vi "Clustering.vi"() -> ()   [LabVIEW 2014]
uses:
  <vilib>/Analysis/Matrix/Datatypes/RealMatrix.ctl
  <vilib>/Analysis/baseanly.llb/Real A x B.vi
  <vilib>/Utility/file.llb/Read From Spreadsheet File (DBL).vi
  <vilib>/Analysis/Matrix/Numeric/Conversions/Matrix To Array - RM.vi
  <vilib>/Utility/file.llb/Read From Spreadsheet File (I64).vi
  <vilib>/Analysis/NI_AALBase.lvlib
  <vilib>/Analysis/Matrix/NI_Matrix.lvlib
panel:
  out "TFD Clustering":i32[](array[numeric])
  out "Centroids of TFD":T1
  out "Centroids of Z (KLD)":T1
  out "Z Clustering (KDL)":i32[](array[numeric])
  out "Centroids of Z (EUC)":T1
  out "Z Clustering (EUC)":i32[](array[numeric])
  out "Centroids of Matrix A":T1
  out "mixing_A Clustering":i32[](array[numeric])
  in  "mixing_A":path
  in  "Selected":path
  in  "inverse_W":path
  in  "STFT":path
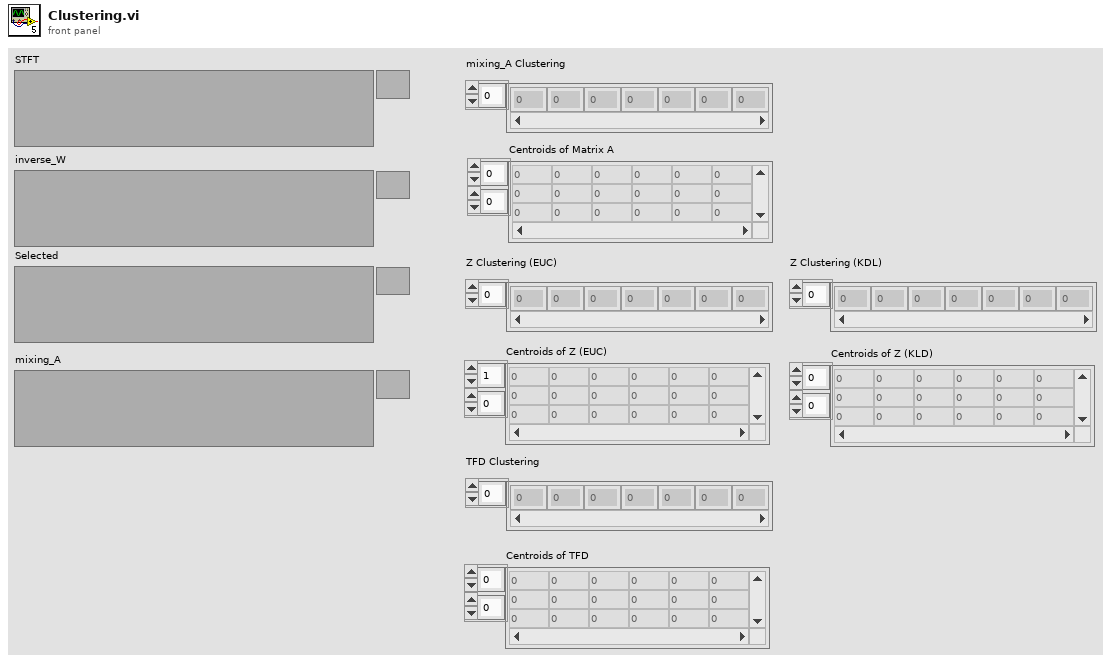
[diagram p1: front panel]
types:
  T1 = typedef "NI_Matrix.lvlib/RealMatrix.ctl" = dbl[][]
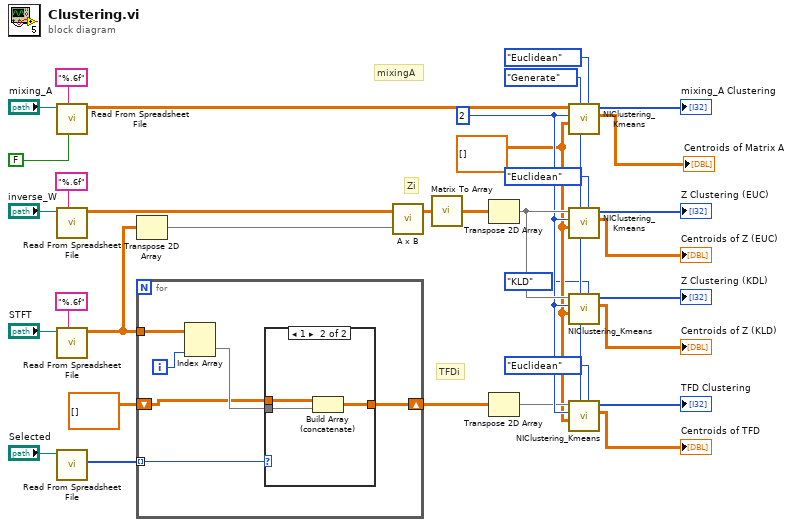
[diagram p0: block diagram]
diagram:
  w13 = dbl[][] [] ("Centroids in")
  w14 = enum16{"Generate", "Input"}."Generate" ("type")
  w16 = 2 ("Classes")
  # "mixingA"
  # "Zi"
  # "TFDi"
  n1 = call-poly <vilib>:"Read From Spreadsheet File.vi"("transpose (no:F)"=FALSE, "format (%.3f)"="%.6f", "file path (dialog if empty)"="mixing_A") -> ("all rows"=w19:dbl[][])  [unwired: 4 in, 4 out]
  n2 = call-poly <vilib>:"Read From Spreadsheet File.vi"("format (%.3f)"="%.6f", "file path (dialog if empty)"="inverse_W") -> ("all rows"=w25:dbl[][])  [unwired: 5 in, 4 out]
  n3 = call-poly <vilib>:"Read From Spreadsheet File.vi"("format (%.3f)"="%.6f", "file path (dialog if empty)"="STFT") -> ("all rows"=w26:dbl[][])  [unwired: 5 in, 4 out]
  n4 = call-poly <vilib>:"Read From Spreadsheet File.vi"("file path (dialog if empty)"="Selected") -> ("first row"=w29:i64[])  [unwired: 6 in, 4 out]
  n5 = Transpose 2D Array(2D array=w26) -> (transposed array=w27:dbl[][])
  n6 = for {
    tunnel: w29 -> [w38] mode=indexing
    tunnel: w26 -> [w40]
    shift-right: [w36] -> w18
    shift-left: dbl[][] [] -> [w35]
    i -> [w39]
    n7 = Index Array(array=w40, index (col)=w39) -> (element=w37:dbl[])  [unwired: 1 in]
    n8 = case shown="1" w38 {
      tunnel: w37 -> [_ w44]
      tunnel: [w41 w43] -> w36
      tunnel: w35 -> [w41 w42]
      frame 0, Default {
      }
      frame 1 {
        n9 = Build Array (concatenate)(w42, w44) -> (w43:dbl[][])
      }
    }
  }
  n10 = call-poly <vilib>:"A x B.vi"("B"=w27, "A"=w25) -> ("A x B"=w21:T1)  [unwired: 1 out]
  n11 = call-poly <vilib>:"Matrix To Array.vi"("Real Matrix"=w21) -> ("Real 2D Array"=w20:dbl[][])
  n12 = Transpose 2D Array(2D array=w20) -> (transposed array=w17:dbl[][])
  n13 = Transpose 2D Array(2D array=w18) -> (transposed array=w15:dbl[][])
  n14 = call "NIClustering_Kmeans.vi"("Enum"=enum16{"KLD", "Euclidean"}."Euclidean", "type"=w14, "Centroids in"=w13, "Classes"=w16, "Data"=w19) -> ("Centroids"=→"Centroids of Matrix A":T1, "Results"=→"mixing_A Clustering":i32[])  [unwired: 4 in, 1 out]
  n15 = call "NIClustering_Kmeans.vi"("Enum"=enum16{"KLD", "Euclidean"}."Euclidean", "type"=w14, "Centroids in"=w13, "Classes"=w16, "Data"=w17) -> ("Centroids"=→"Centroids of Z (EUC)":T1, "Results"=→"Z Clustering (EUC)":i32[])  [unwired: 4 in, 1 out]
  n16 = call "NIClustering_Kmeans.vi"("Enum"=enum16{"KLD", "Euclidean"}."KLD", "type"=w14, "Centroids in"=w13, "Classes"=w16, "Data"=w17) -> ("Centroids"=→"Centroids of Z (KLD)":T1, "Results"=→"Z Clustering (KDL)":i32[])  [unwired: 4 in, 1 out]
  n17 = call "NIClustering_Kmeans.vi"("Enum"=enum16{"KLD", "Euclidean"}."Euclidean", "type"=w14, "Centroids in"=w13, "Classes"=w16, "Data"=w15) -> ("Centroids"=→"Centroids of TFD":T1, "Results"=→"TFD Clustering":i32[])  [unwired: 4 in, 1 out]
